vi "Parse TSF.vi"(8 "error in (no error)":errorcluster, 11 "TSF Parser in":refnum<class "TSF Parser.lvclass">) -> (0 "error out":errorcluster, 3 "TSF Parser out":refnum<class "TSF Parser.lvclass">)   [LabVIEW 2016, in "TSF Parser.lvlib" / "TSF Parser.lvclass"]
uses:
  TSF Parser.lvclass
  <vilib>/Utility/NIReport.llb/NI_report.lvclass
  <vilib>/addons/_office/NI_ReportGenerationToolkit.lvlib
  <vilib>/Utility/NIReport.llb/Excel/NI_Excel.lvclass
  <vilib>/addons/_office/excel.llb/Excel Get Data ([str]).vi
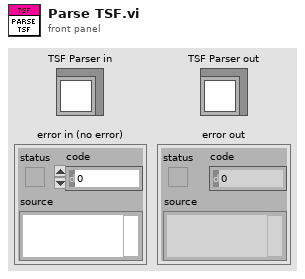
[diagram p1: front panel]
types:
  T1 = enum16{"Standard Report", "HTML", "Word", "Excel"}
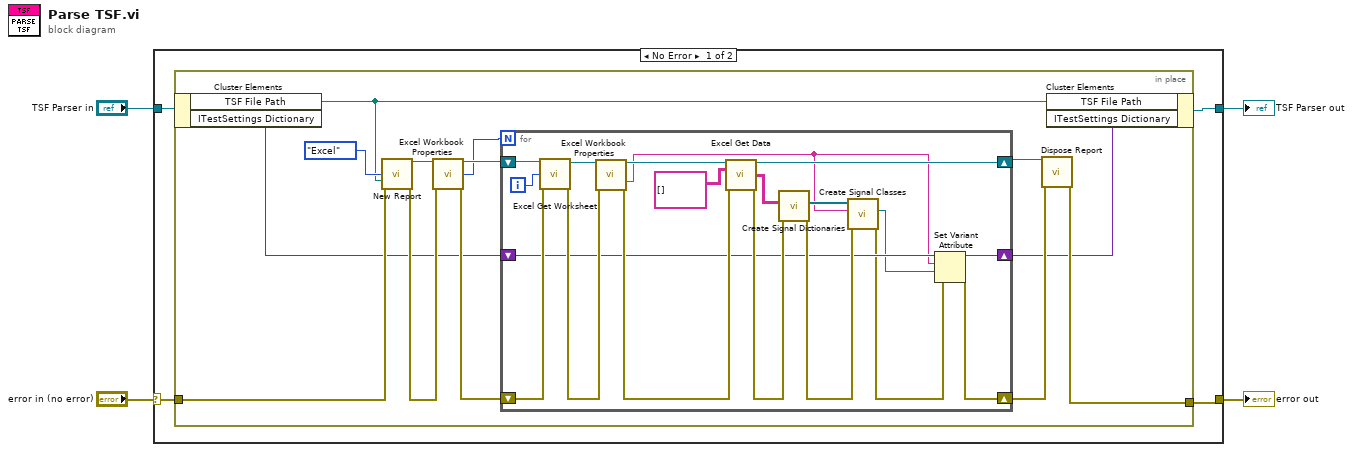
[diagram p0: block diagram]
diagram:
  n1 = case shown="No Error" "error in (no error)" {
    selector: "error in (no error)" -> [w7 w42]
    tunnel: [w5 w42] -> w3
    tunnel: [w6 w41] -> w1
    tunnel: "TSF Parser in" -> [w8 w41]
    frame No Error {
      n2 = in-place {
        in-place-border: w7 -> [w21]
        in-place-border: [w12] -> w5
        n3 = in-place-cluster #1(w8) -> ("TSF File Path"=w11:path, "ITestSettings Dictionary"=w10:variant)
        n4 = call <vilib>:"New Report.vi"("report type"=T1."Excel", "template (empty)"=w11, "error in (no error)"=w21) -> ("report out"=w19:refnum<class "NI_report.lvclass">, "error out"=w18:errorcluster)  [unwired: 11 in]
        n5 = call <vilib>:"Excel Workbook Properties.vi"("report in"=w19, "error in (no error)"=w18) -> ("report out"=w17:refnum<class "NI_report.lvclass">, "worksheets count"=w16:i32, "error out"=w15:errorcluster)  [unwired: 10 in, 1 out]
        n6 = for {
          N: w16 -> [_]
          shift-right: [w24] -> w13
          shift-left: w15 -> [w38]
          shift-right: [w33] -> w14
          shift-left: w17 -> [w40]
          shift-right: [w23] -> w9
          shift-left: w10 -> [w27]
          i -> [w39]
          n7 = call <vilib>:"Excel Get Worksheet.vi"("report in"=w40, "worksheet index (0)"=w39, "error in (no error)"=w38) -> ("report out"=w37:refnum<class "NI_report.lvclass">, "error out"=w36:errorcluster)  [unwired: 11 in]
          n8 = call <vilib>:"Excel Workbook Properties.vi"("report in"=w37, "error in (no error)"=w36) -> ("report out"=w35:refnum<class "NI_report.lvclass">, "current worksheet name"=w22:string, "error out"=w32:errorcluster)  [unwired: 10 in, 1 out]
          n9 = call-poly <vilib>:"Excel Get Data.vi"("report in"=w35, "data type"=string[][] [], "error in (no error)"=w32) -> ("report out"=w33:refnum<class "NI_report.lvclass">, "data"=w31:string[][], "error out"=w30:errorcluster)  [unwired: 10 in]
          n10 = call "Create Signal Dictionaries.vi"("error In"=w30, "Raw Data"=w31) -> ("Error Out"=w28:errorcluster, "Parameter Array Out"=w29:refnum<class "String Database.lvclass">[])  [unwired: 8 in]
          n11 = call "Create Signal Classes.vi"("error in (no error)"=w28, "TSF Tab"=w22, "Parameter Array In"=w29) -> ("error out"=w25:errorcluster, "ITestSettings out"=w26:refnum<class "ITestSettings.lvclass">)  [unwired: 7 in]
          n12 = Set Variant Attribute(Variant=w27, name=w22, value=w26, error in=w25) -> (Variant out=w23:variant, error out=w24:errorcluster)  [unwired: 1 out]
        }
        n13 = call-dynamic "Dispose Report.vi"("report in"=w14, "error in (no error)"=w13) -> ("error out"=w12:errorcluster)  [unwired: 13 in]
        n14 = in-place-cluster #1("TSF File Path"=w11, "ITestSettings Dictionary"=w9) -> (w6:refnum<class "TSF Parser.lvclass">)
      }
    }
    frame Error {
    }
  }
  "error out" <- w3
  "TSF Parser out" <- w1
